vi "Oxford GPIB transaction.vi"(2 "Command String":string, 3 "GPIB Address":refnum<visa-resource-name>) -> (0 "Stop":bool, 1 "Measurement":dbl[](array[numeric]) format="%.2e")   [LabVIEW 2019]
doc: "This is a modified version, to deal with Oxford's use of carriage returns rather than AOI\n\nThis VI reads a single reading from a Keithley 2001 multimeter. The stop boolean is always false. If no reading is obtained a single zero is returned.\nScott Hannahs, NHMFL-FSU, Nov 1993"
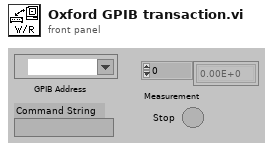
[diagram p1: front panel]
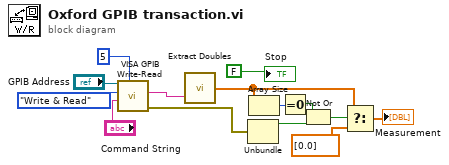
[diagram p0: block diagram]
diagram:
  n1 = call "VISA GPIB Write-Read.vi"("Wait (ms)"=u32 5 ("wait (mS)"), "Command"="Command String", "Action"=enum16{"Write", "Read", "Write & Read"}."Write & Read", "VISA resource name"="GPIB Address") -> ("error out"=w3:errorcluster, "String Returned"=w4:string)  [unwired: 4 in, 2 out]
  n2 = call "Extract Doubles.vi"("String"=w4) -> ("Data"=w9:dbl[])  [unwired: 1 in]
  n3 = Unbundle(w3) -> ("status"=w11:bool)  [unwired: 2 out]
  n4 = Array Size(array=w9) -> (size(s)=w13:i32)
  n5 = Equal To 0?(x=w13) -> (x = 0?=w12:bool)
  n6 = Not Or(1:w11, 2:w12) -> (0:w10:bool)
  n7 = Select(t=w9, s=w10, f=dbl[] [0.0]) -> (s? t:f=→"Measurement":dbl[])
  "Stop" <- FALSE
